vi "Digitizer Analyze_SNRPhaseNoise.vi"(4 "frequency range":T2={"start frequency"=-1.0, "stop frequency"=-1.0}, 5 "band":T1 {"stop frequency (Hz)" format="%.2f"; "start frequency (Hz)" format="%.2f"}, 6 "Pins":string[](array[string])=["Xout"], 7 "error in":errorcluster, 8 "Published Data Id":string[](array[string]), 9 "Waveform Data In":waveform(dbl)[](array[waveform])=[{"t0"=timestamp(3637030365.2340937 s since 1904-01-01), "dt"=3.3333333333333334e-08, "Y"=array[5343 elements]}, {"t0"=timestamp(3637030365.2340937 s since 1904-01-01), "dt"=3.3333333333333334e-08, "Y"=array[5343 elements]}], 10 "Semiconductor Module Context":T3) -> (0 "error out":errorcluster)   [LabVIEW 2014]
doc: "Example: Measurement Library\n\nRecommended Input Signal: 100 kHz, 2 Vpp, sine wave\n\nDevices Supported: Refer to NI Example Finders\n\nLabVIEW Description:\n\nThis example illustrates fetching scalar measurements from NI-SCOPE, such as period and rise time calculations. \n\nSome common horizontal and vertical parameters are configured for the oscilloscope. The property node is used to set the reference level units, and the low, middle and high reference levels. For more information about measurement library parameters, see the NI-SCOPE VI Reference Help file. \n\nAfter the Read VI is called to acquire a waveform, the Fetch Measurement Stats VI is used to perform the desired scalar measurement analysis on the waveform. NI-SCOPE keeps a history of each measurement's results, which allows it to retrieve the statistics computed over multiple acquisitions. These statistics include the mean, standard deviation, min, max and number of acquisitions used in the statistics. The statistics are updated once per acquisition when the measurement is fetched. The Clear Stats VI clears this history."
uses:
  <vilib>/NI_TestStand_SemiconductorModule/NI_TestStand_Semiconductor_Module.lvlibp/PinMap/General/SemiconductorModuleContext.ctl
  <vilib>/NI_TestStand_SemiconductorModule/NI_TestStand_Semiconductor_Module.lvlibp/PinMap/General/NIInstrumentTypeIDs.ctl
  <vilib>/addons/_NISVFA/_Shared subVIs/Controls/svc_Window.ctl
  <vilib>/addons/_NISVFA/_Baseband FFT/SVFA FFT Spectrum (Complex) (1 Ch).vi
  <vilib>/addons/_NISVFA/_Spectrum Processing/SVFA Unit Conversion (Complex) (1 Ch).vi
  <vilib>/NI_TestStand_SemiconductorModule/NI_TestStand_Semiconductor_Module.lvlibp/PinMap/General/Publish/PublishDataDoubleFunctionalTest.vi
  <vilib>/NI_TestStand_SemiconductorModule/NI_TestStand_Semiconductor_Module.lvlibp
panel:
  out "Frequency (Hz)":dbl format="%.2f"
  out "SNR (dB)":dbl format="%.2f"
  out "Power (dBm)":dbl
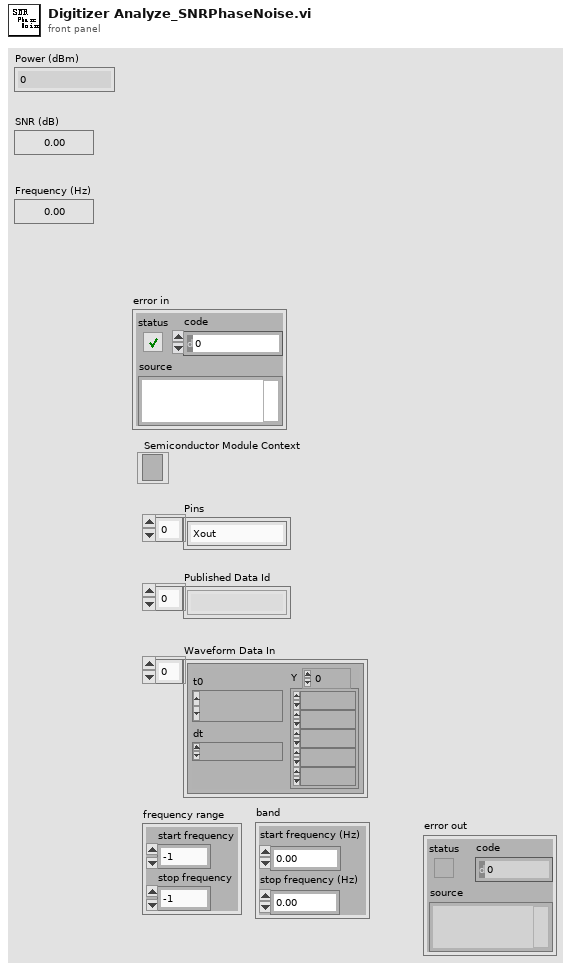
[diagram p1: front panel]
types:
  T1 = cluster{"start frequency (Hz)":dbl, "stop frequency (Hz)":dbl}
  T2 = cluster{"start frequency":dbl, "stop frequency":dbl}
  T3 = typedef "NI_TestStand_Semiconductor_Module.lvlibp/SemiconductorModuleContext.ctl" = refnum<k7>
  T4 = typedef "svc_Window.ctl" = u32
  T5 = typedef "NI_TestStand_Semiconductor_Module.lvlibp/NIInstrumentTypeIDs.ctl" = string
  T6 = cluster{"linear/dB":enum16{"no change", "linear", "dB"}, "dB reference (0: no change)":dbl, "power/magnitude":enum16{"no change", "power", "magnitude"}, "view":enum16{"no change", "rms", "peak", "peak-peak"}}
  T7 = typedef "svc_Spectrum Info.ctl" = cluster{"channel name":string, "description":string, "x-axis units":T8, "spectral info":cluster{"spectrum type":T9, "linear/dB":enum16{"linear", "dB"}, "window":u16, "window size":i32, "FFT size":i32}, "engineering units":T10, "custom label":string, "dB reference [EU]":dbl, "peak units":enum16{"rms", "peak", "peak-peak"}, "weighting filter":T11, "spectral density?":bool, "unit label":string, "spectrum skewed?":bool, "complimentary spectrum units":T12}
  T8 = typedef "svc_X-Axis Units.ctl" = u16
  T9 = typedef "svc_Spectrum Type.ctl" = enum16{"FFT Spectrum [complex]", "Amplitude [Magnitude]", "Power [Magnitude^2]", "Cross Spectrum [complex]", "Frequency Response [Complex]"}
  T10 = typedef "svc_Engineering Units Text Ring.ctl" = u16
  T11 = typedef "svc_Weighting Filter Text Ring.ctl" = u16
  T12 = typedef "svc_Complimentary Spectrum Units.ctl" = enum16{"none", "radians", "degrees", "cycles", "imaginary"}
  T13 = cluster{"complex spectrum response":cluster{"f0":dbl, "df":dbl, "complex spectrum":cdb[]}, "spectrum info":T7}
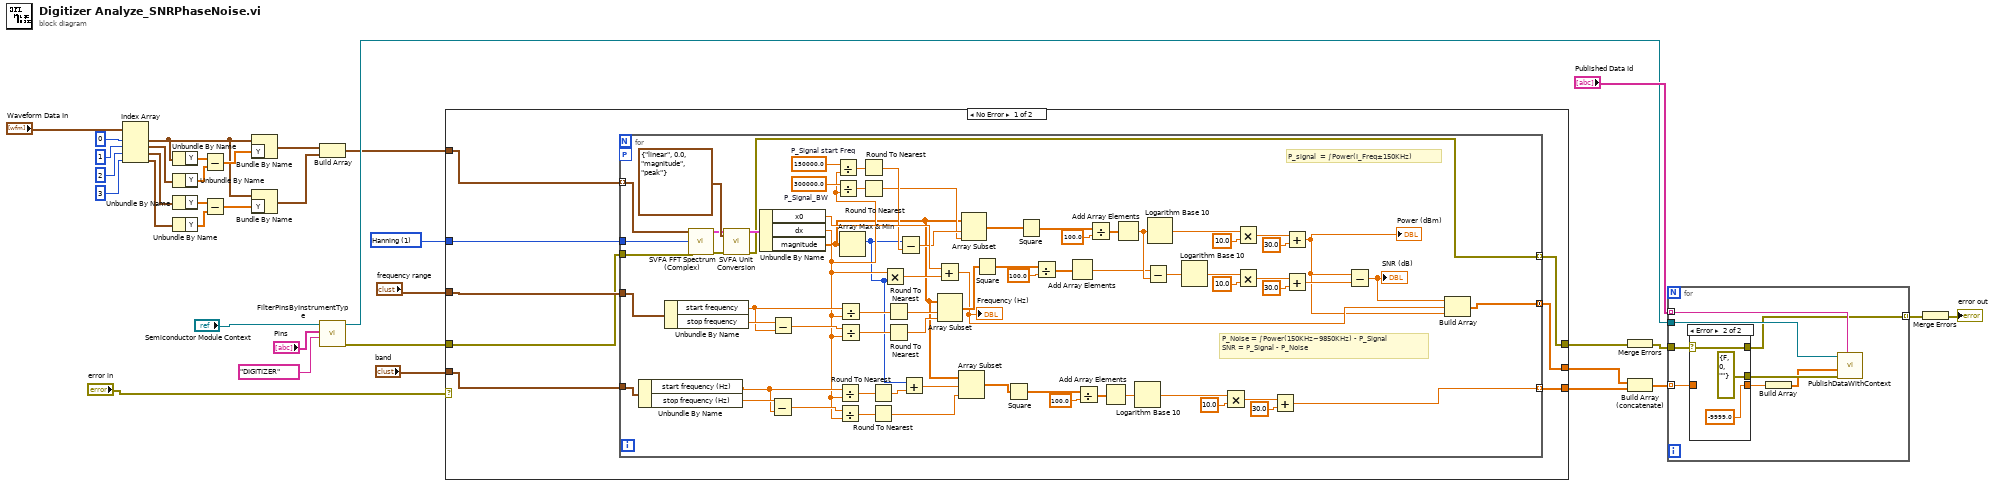
[diagram p0: block diagram]
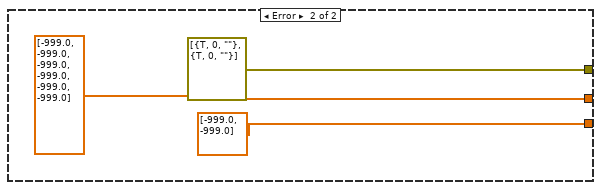
[diagram p2: hidden frame]
diagram:
  w31 = T4 1 items=["None"=0, "Hanning"=1, "Hamming"=2, "Blackman-Harris"=3, "Exact Blackman"=4, "Blackman"=5, "Flat Top"=6, "4 Term B-Harris "=7, "7 Term B-Harris"=8, "Low Sidelobe"=9, "Force"=64, "Exponential"=65, "Blackman Nuttall"=11, "Triangle"=30, "Bartlett-Hanning"=31, "Bohman"=32, "Parzen"=33, "Welch"=34, "Kaiser"=60, "Dolph-Chebyshev"=61, "Gaussian"=62] ("window")
  n1 = Index Array(array="Waveform Data In", index #1=0 ("index"), index #2=1 ("index"), index #3=2 ("index"), index #4=3 ("index")) -> (element #1=w16:waveform(dbl), element #2=w24:waveform(dbl), element #3=w23:waveform(dbl), element #4=w22:waveform(dbl))
  n2 = Unbundle By Name(w16) -> ("Y"=w28:dbl[])
  n3 = Unbundle By Name(w24) -> ("Y"=w27:dbl[])
  n4 = Unbundle By Name(w23) -> ("Y"=w19:dbl[])
  n5 = Unbundle By Name(w22) -> ("Y"=w18:dbl[])
  n6 = Subtract(x=w28, y=w27) -> (x-y=w32:dbl[])
  n7 = Subtract(x=w19, y=w18) -> (x-y=w17:dbl[])
  n8 = Bundle By Name(cluster=w16, "Y"=w32) -> (w15:waveform(dbl))
  n9 = Bundle By Name(cluster=w16, "Y"=w17) -> (w14:waveform(dbl))
  n10 = Build Array(w15, w14) -> (w6:waveform(dbl)[])
  n11 = call <vilib>:"FilterPinsByInstrumentType.vi"("Instrument Type Id"=T5 "DIGITIZER", "Pins"="Pins", "Semiconductor Module Context"="Semiconductor Module Context") -> ("error out"=w5:errorcluster, "Semiconductor Module Context Out"=w25:T3)  [unwired: 6 in, 1 out]
  n12 = case shown="No Error" "error in" {
    tunnel: w31 -> [w41 _]
    tunnel: [w37 dbl[] [-999.0, -999.0, -999.0, -999.0, -999.0, -999.0]] -> w11
    tunnel: [w36 errorcluster[] [{"status"=TRUE, "code"=0, "source"=""}, {"status"=TRUE, "code"=0, "source"=""}]] -> w9
    tunnel: w6 -> [w42 _]
    tunnel: w5 -> [w40 _]
    tunnel: "frequency range" -> [w43 _]
    tunnel: "band" -> [w39 _]
    tunnel: [w38 dbl[] [-999.0, -999.0]] -> w2
    frame No Error {
      n13 = for {
        tunnel: w42 -> [w83] mode=indexing
        tunnel: w41 -> [w84]
        tunnel: [w114] -> w37 mode=concatenating
        tunnel: w43 -> [w79]
        workers-P: _ -> [_]
        tunnel: w40 -> [w85]
        tunnel: [w86] -> w36 mode=indexing
        tunnel: w39 -> [w65]
        tunnel: [w45] -> w38 mode=indexing
        w68 = 300000.0  # P_Signal_BW
        w69 = 150000.0  # P_Signal start Freq
        # "P_Noise = ∫Power(150KHz~9850KHz) - P_Signal\nSNR = P_Signal - P_Noise"
        # "P_signal  = ∫Power(I_Freq±150KHz)"
        n14 = Unbundle By Name(w65) -> ("start frequency (Hz)"=w60:dbl, "stop frequency (Hz)"=w61:dbl)
        n15 = Unbundle By Name(w79) -> ("start frequency"=w75:dbl, "stop frequency"=w76:dbl)
        n16 = call-poly <vilib>:"SVFA FFT Spectrum (Complex).vi"("scaled signal [EU]"=w83, "window"=w84, "error in"=w85) -> ("complex spectrum"=w87:T13, "error out"=w88:errorcluster)  [unwired: 13 in, 2 out]
        n17 = call-poly <vilib>:"SVFA Unit Conversion.vi"("complex spectrum"=w87, "desired scaling"=T6 {"linear/dB"=enum."linear", "dB reference (0: no change)"=0.0, "power/magnitude"=enum."magnitude", "view"=enum."peak"}, "error in (no error)"=w88) -> ("converted spectrum"=w90:cluster{"x0":dbl, "dx":dbl, "magnitude":dbl[]}, "error out"=w86:errorcluster)  [unwired: 11 in, 4 out]
        n18 = Unbundle By Name(w90) -> ("x0"=w100:dbl, "dx"=w59:dbl, "magnitude"=w58:dbl[])
        n19 = Subtract(x=w61, y=w60) -> (x-y=w63:dbl)
        n20 = Subtract(x=w76, y=w75) -> (x-y=w74:dbl)
        n21 = Divide(x=w69, y=w59) -> (x/y=w71:dbl)
        n22 = Divide(x=w68, y=w59) -> (x/y=w70:dbl)
        n23 = Divide(x=w60, y=w59) -> (x/y=w64:dbl)
        n24 = Divide(x=w63, y=w59) -> (x/y=w62:dbl)
        n25 = Divide(x=w75, y=w59) -> (x/y=w78:dbl)
        n26 = Divide(x=w74, y=w59) -> (x/y=w73:dbl)
        n27 = Array Max & Min(array=w58) -> (max index (indices)=w55:i32)  [unwired: 3 out]
        n28 = Round To Nearest(number=w71) -> (nearest integer value=w67:dbl)
        n29 = Round To Nearest(number=w70) -> (nearest integer value=w66:dbl)
        n30 = Round To Nearest(number=w64) -> (nearest integer value=w57:dbl)
        n31 = Round To Nearest(number=w62) -> (nearest integer value=w44:dbl)
        n32 = Multiply(x=w59, y=w55) -> (x*y=w101:dbl)
        n33 = Round To Nearest(number=w78) -> (nearest integer value=w77:dbl)
        n34 = Round To Nearest(number=w73) -> (nearest integer value=w72:dbl)
        n35 = Subtract(x=w55, y=w67) -> (x-y=w91:dbl)
        n36 = Add(x=w55, y=w57) -> (x+y=w56:dbl)
        n37 = Add(x=w100, y=w101) -> (x+y=w81:dbl)
        "Frequency (Hz)" <- w81
        n38 = Array Subset(array=w58, index=w77, length=w72) -> (w109:dbl[])
        n39 = Array Subset(array=w58, index=w56, length=w44) -> (w46:dbl[])
        n40 = Array Subset(array=w58, index=w91, length=w66) -> (w92:dbl[])
        n41 = Square(x=w109) -> (x^2=w102:dbl[])
        n42 = Square(x=w46) -> (x^2=w47:dbl[])
        n43 = Square(x=w92) -> (x^2=w93:dbl[])
        n44 = Divide(x=w102, y=100.0) -> (x/y=w104:dbl[])
        n45 = Add Array Elements(numeric array=w104) -> (sum=w110:dbl)
        n46 = Divide(x=w47, y=100.0) -> (x/y=w49:dbl[])
        n47 = Divide(x=w93, y=100.0) -> (x/y=w95:dbl[])
        n48 = Add Array Elements(numeric array=w49) -> (sum=w54:dbl)
        n49 = Add Array Elements(numeric array=w95) -> (sum=w111:dbl)
        n50 = Logarithm Base 10(1:w54) -> (0:w50:dbl)
        n51 = Subtract(x=w110, y=w111) -> (x-y=w112:dbl)
        n52 = Logarithm Base 10(1:w111) -> (0:w96:dbl)
        n53 = Logarithm Base 10(1:w112) -> (0:w105:dbl)
        n54 = Multiply(x=w50, y=10.0) -> (x*y=w52:dbl)
        n55 = Multiply(x=w96, y=10.0) -> (x*y=w98:dbl)
        n56 = Multiply(x=w105, y=10.0) -> (x*y=w107:dbl)
        n57 = Add(x=w52, y=30.0) -> (x+y=w45:dbl)
        n58 = Add(x=w98, y=30.0) -> (x+y=w80:dbl)
        "Power (dBm)" <- w80
        n59 = Add(x=w107, y=30.0) -> (x+y=w113:dbl)
        n60 = Subtract(x=w80, y=w113) -> (x-y=w82:dbl)
        "SNR (dB)" <- w82
        n61 = Build Array(w82, w81, w80) -> (w114:dbl[])
      }
    }
    frame Error {
    }
  }
  n62 = Merge Errors(w9) -> (w8:errorcluster)
  n63 = Build Array (concatenate)(w11, w2) -> (w10:dbl[])
  n64 = for {
    tunnel: "Published Data Id" -> [w125] mode=indexing
    tunnel: w10 -> [w122] mode=indexing
    tunnel: w25 -> [w124]
    tunnel: w8 -> [w123]
    tunnel: [w119] -> w13 mode=indexing
    n65 = case shown="Error" w123 {
      selector: w123 -> [w126 w129]
      tunnel: w122 -> [w127 _]
      tunnel: [w127 -9999.0 ("detected fundamental\nfrequency [Hz]")] -> w121
      tunnel: [w126 errorcluster {"status"=FALSE, "code"=0, "source"=""} ("error IO")] -> w120
      tunnel: [w126 w129] -> w119
      frame No Error {
      }
      frame Error {
      }
    }
    n66 = Build Array(w121) -> (w118:dbl[])
    n67 = call-poly <vilib>:"PublishDataWithContext.vi"("Published Data Id"=w125, "error in (no error)"=w120, "Data In"=w118, "Semiconductor Module Context"=w124) -> ()  [unwired: 6 in, 2 out]
  }
  n68 = Merge Errors(w13) -> (→"error out":errorcluster)
